vi "OE2031&OE2041_Configure Channel Out.vi"(7 "OE2041_Configure Channel Out":T1={"parameter"=0, "Speed"=0, "Offset(%)"=0.0, "Expand"=1.0, "AUX OUT"=1.0, "Channel"=0} {"Channel" items=["CH1", "CH2", "CH3", "CH4"]; "AUX OUT" min=-10.0 max=10.0 format="%#.3g"; "Expand" min=1.0 max=256.0 format="%#_3g"; "Offset(%)" min=-100.0 max=100.0 format="%#_5g"; "Speed" items=["Slow", "Fast"]; "parameter" items=["AUXOUT", "X", "Y", "R", "Theta", "Xh1", "Yh1", "Rh1", "Theta h1", "Xh2", "Yh2", "Rh2", "Theta h2", "Xh3", "Yh3", "Rh3", "Theta h3", "X_Noise", "Y_Noise", "Frequency", "AUX-IN1", "AUX-IN2", "AUX-IN3", "AUX-IN4"]}, 8 "Error in (no error)":errorcluster caption="error out（no error）", 9 "Remote Mode":u16(ring) items=["USB"=0, "RS232"=1, "Ethernet"=3], 10 "Connection ID in":refnum<k5>, 11 "VISA resource name":refnum<visa-resource-name>) -> (0 "Error out":errorcluster caption="error out", 1 "Output String":string, 2 "Connection ID out":refnum<k5>, 3 "VISA resource  out":refnum<visa-resource-name>)   [LabVIEW 2011]
panel:
  out "Channel":u16
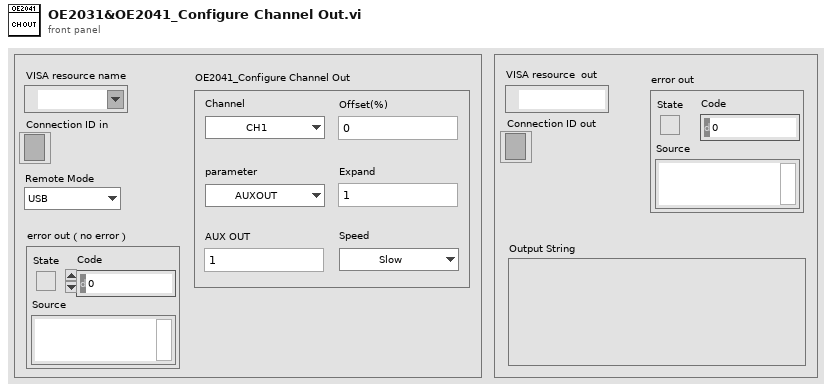
[diagram p1: front panel]
types:
  T1 = cluster{"parameter":u16, "Speed":u16, "Offset(%)":dbl, "Expand":dbl, "AUX OUT":dbl, "Channel":u16}
  T2 = enum16{"ISRC", "IGND", "ICPL", "ILIN", "PHAS", "FMOD", "RSLP", "FREQ", "SWPT", "SLLM", "SULM", "SSLL", "SSLG", "STLM", "SWRM", "IRNG", "SENS", "RMOD", "OFLT", "OFSL", "SYNC", "DMOD", "HARM", "DARB", "SWVT", "SLVL", "SVLL", "SVUL", "SVSL", "SVSG", "SVTM", "SVRM", "RALL", "SNAP", "OUTP", "OAUX", "COUT", "CAUX", "COFP", "CEXP", "FPOP", "OEXP", "*IDN", "*RST", "OVLD", "INOV", "GNOV", "*PLL", "SSET", "RSET", "AGAN", "APHS", "ARSV", "ASCL", "EQCD", "EQCS", "SPED", "SRAT", "SLEN", "SSLE", "STRG", "SPRM", "STRD", "PAUS", "REST", "SPTS", "TRCA", "TEMP", "RSTU", "IHNZ", "DEQU", "SADD", "ARNG", "CSPE", "ISRCD", "IGNDD", "ICPLD", "ILIND", "PHASD", "FMODD", "RSLPD", "FREQD", "SWPTD", "SLLMD", "SULMD", "SSLLD", "SSLGD", "STLMD", "SWRMD", "SENSD", "RMODD", "OFLTD", "OFSLD", "SYNCD", "HARMD", "EQCDD", "EQCSD", "SNAPD", "OUTPD", "SWVTD", "SLVLD", "SVLLD", "SVULD", "SVSLD", "SVSGD", "SVTMD", "SVRMD", "SVDCD", "ARSVD", "AGAND", "APHSD", "ASCLD", "FPOPD", "CAUXD", "OEXPD", "SPEDD", "SRATD", "SLEND", "SSLED", "STRGD", "SPRMD", "STRDD", "PAUSD", "RESTD", "SPTSD", "TRCAD", "*IDND", "*RSTD", "INOVD", "GNOVD", "*PLLD", "SSETD", "RSETD", "RALLD"}
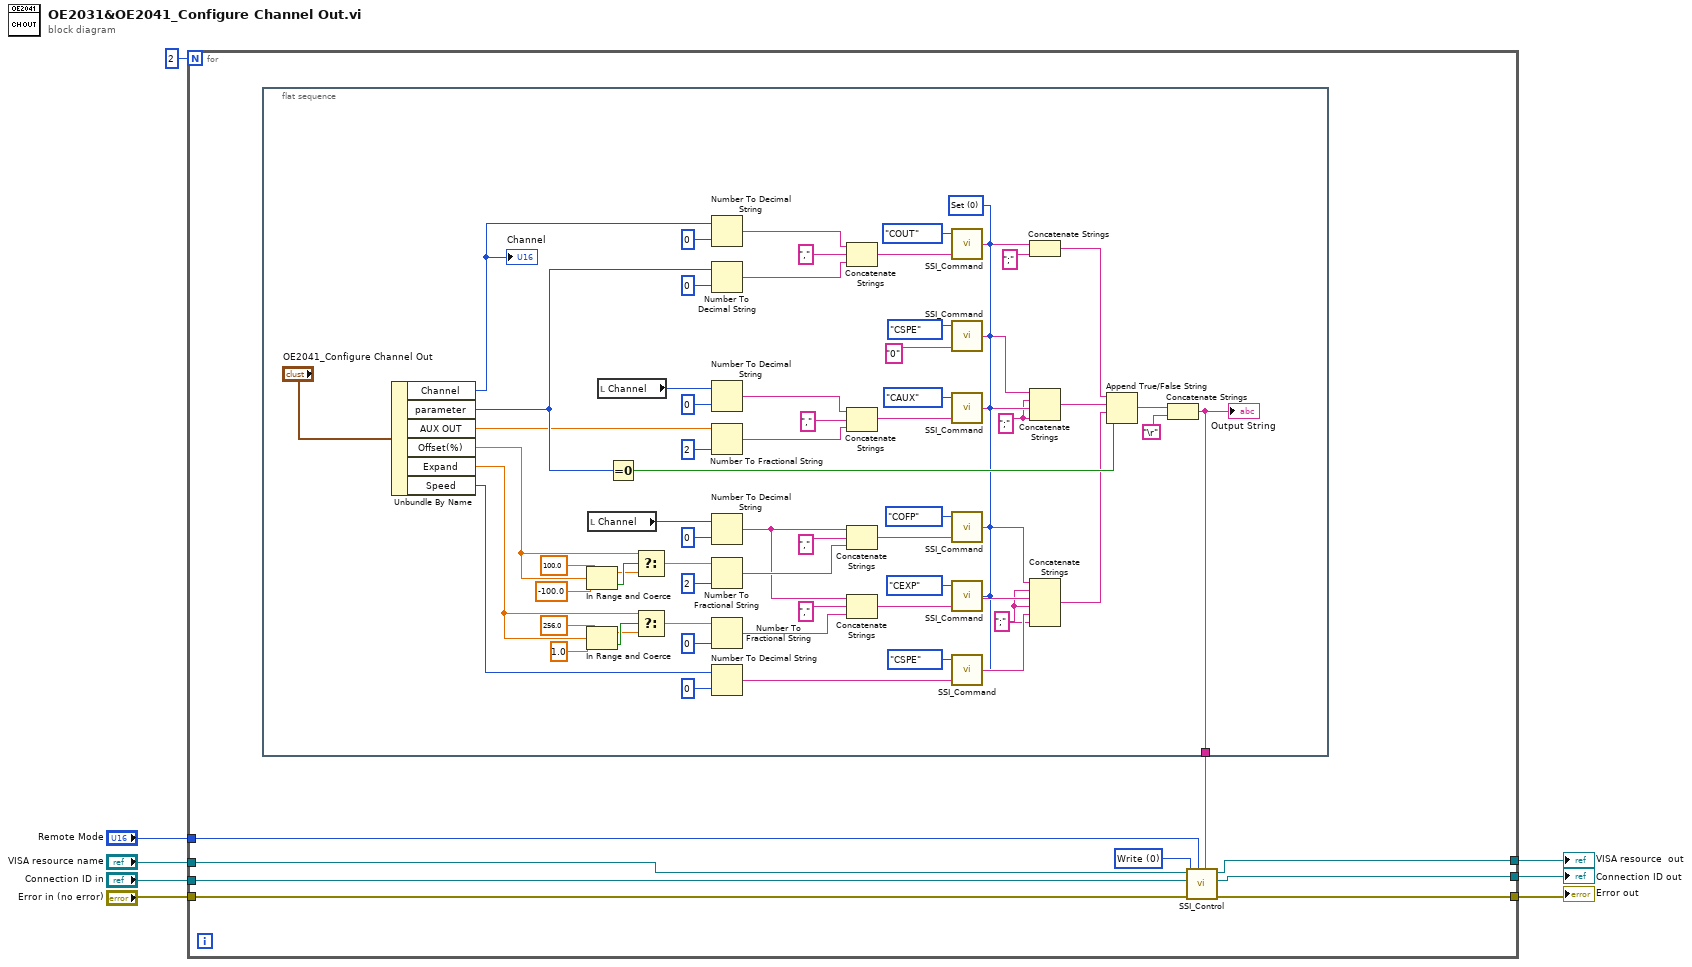
[diagram p0: block diagram]
diagram:
  n1 = for {
    N: 2 -> [_]
    tunnel: "Connection ID in" -> [w15]
    tunnel: "Error in (no error)" -> [w14]
    tunnel: "VISA resource name" -> [w13]
    tunnel: "Remote Mode" -> [w12]
    tunnel: [w11] -> w3
    tunnel: [w10] -> w2
    tunnel: [w9] -> w1
    w17 = u16 0 items=["Write", "Read"] ("Control")
    n2 = flat-sequence {
      tunnel: [w35] -> w16
      frame #0 {
        w36 = ";" ("字符串")
        w21 = ";" ("替换字符串(\"\")")
        w22 = u16 0 items=["Set", "Query"] ("Opera")
        n3 = Unbundle By Name("OE2041_Configure Channel Out") -> ("Channel"=w64:u16, "parameter"=w57:u16, "AUX OUT"=w48:dbl, "Offset(%)"=w34:dbl, "Expand"=w33:dbl, "Speed"=w52:u16)
        "Channel" <- w64
        n4 = In Range and Coerce(upper limit=100.0 ("上限"), x=w34, lower limit=-100.0 ("下限")) -> (coerced(x)=w72:dbl, In Range?=w73:bool)
        n5 = In Range and Coerce(upper limit=256.0 ("上限"), x=w33, lower limit=1.0 ("下限")) -> (coerced(x)=w77:dbl, In Range?=w78:bool)
        n6 = local read "Channel"() -> (w20:u16)
        n7 = local read "Channel"() -> (w27:u16)
        n8 = Equal To 0?(x=w57) -> (x = 0?=w56:bool)
        n9 = Select(t=w34, s=w73, f=w72) -> (s? t:f=w66:dbl)
        n10 = Select(t=w33, s=w78, f=w77) -> (s? t:f=w74:dbl)
        n11 = Number To Decimal String(number=w64, width (-)=i16 0 ("精度(6)")) -> (decimal integer string=w61:string)
        n12 = Number To Decimal String(number=w57, width (-)=i16 0 ("精度(6)")) -> (decimal integer string=w60:string)
        n13 = Number To Decimal String(number=w27, width (-)=i16 0 ("精度(6)")) -> (decimal integer string=w25:string)
        n14 = Number To Fractional String(number=w48, precision (6)=i16 2 ("精度(6)")) -> (F-format string=w31:string)  [unwired: 2 in]
        n15 = Number To Decimal String(number=w20, width (-)=i16 0 ("精度(6)")) -> (decimal integer string=w29:string)
        n16 = Number To Fractional String(number=w66, precision (6)=i16 2 ("精度(6)")) -> (F-format string=w46:string)  [unwired: 2 in]
        n17 = Number To Fractional String(number=w74, precision (6)=i16 0 ("精度(6)")) -> (F-format string=w42:string)  [unwired: 2 in]
        n18 = Number To Decimal String(number=w52, width (-)=i16 0 ("精度(6)")) -> (decimal integer string=w24:string)
        n19 = Concatenate Strings(w61, "," ("字符串"), w60) -> (w62:string)
        n20 = Concatenate Strings(w25, "," ("字符串"), w31) -> (w30:string)
        n21 = Concatenate Strings(w29, "," ("字符串"), w46) -> (w47:string)
        n22 = Concatenate Strings(w29, "," ("字符串"), w42) -> (w44:string)
        n23 = call "SSI_Command.vi"("Opera"=w22, "Paramter"=w62, "Command Type"=T2."COUT") -> ("Output string"=w80:string)  [unwired: 1 in]
        n24 = call "SSI_Command.vi"("Opera"=w22, "Paramter"="0" ("字符串"), "Command Type"=T2."CSPE") -> ("Output string"=w23:string)  [unwired: 1 in]
        n25 = call "SSI_Command.vi"("Opera"=w22, "Paramter"=w30, "Command Type"=T2."CAUX") -> ("Output string"=w82:string)  [unwired: 1 in]
        n26 = call "SSI_Command.vi"("Opera"=w22, "Paramter"=w47, "Command Type"=T2."COFP") -> ("Output string"=w41:string)  [unwired: 1 in]
        n27 = call "SSI_Command.vi"("Opera"=w22, "Paramter"=w44, "Command Type"=T2."CEXP") -> ("Output string"=w79:string)  [unwired: 1 in]
        n28 = call "SSI_Command.vi"("Opera"=w22, "Paramter"=w24, "Command Type"=T2."CSPE") -> ("Output string"=w37:string)  [unwired: 1 in]
        n29 = Concatenate Strings(w80, ";" ("替换字符串(\"\")")) -> (w19:string)
        n30 = Concatenate Strings(w23, w21, w82, w21) -> (w50:string)
        n31 = Concatenate Strings(w41, w36, w79, w36, w37, w36) -> (w38:string)
        n32 = Append True/False String(1:w56, 2:w38, 3:w50, 4:w19) -> (0:w39:string)
        n33 = Concatenate Strings(w39, "\r") -> (w35:string)
        "Output String" <- w35
      }
    }
    n34 = call "SSI_Control.vi"("Write Buffer"=w16, "Remote Mode"=w12, "Error in (no error)"=w14, "Control"=w17, "Connection ID in"=w15, "VISA resource name"=w13) -> ("Error out"=w9:errorcluster, "Connection ID out"=w10:refnum<k5>, "VISA resource  out"=w11:refnum<visa-resource-name>)  [unwired: 2 in, 1 out]
  }
  "Error out" <- w1
  "Connection ID out" <- w2
  "VISA resource  out" <- w3
